vi "CRYPIC PreLoad.vi"(9 "sVIName":string) -> (1 "sVITitle_Out":string)   [LabVIEW 2013]
uses:
  DataView/VIEW/CRYView Global.vi
  CRYMain Sub Window Global.vi
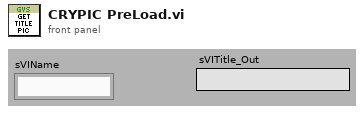
[diagram p1: front panel]
types:
  T1 = cluster{"sAction":string, "sType":string, "sQueueName":string, "sGraphName":string, "sData":string, "nData":i32, "pVIRef":refnum<vi>, "pSPRef":refnum<vi>}
  T2 = typedef "LVRectTypeDef.ctl" = cluster{"Left":i16, "Top":i16, "Right":i16, "Bottom":i16}
  T3 = cluster{"nType":i32, "nParent":i32, "pVIW":refnum<vi>, "pSPW":refnum<vi>, "nTypeF":i32, "pVIF":refnum<vi>, "pSPF":refnum<vi>, "nIDSpliter":i32, "nProperty":i32, "Bound":T2, "nID":i32, "nData":i32, "sData":string, "pWVI":refnum<vi>, "sTitle":string, "cPages":cluster{"nPage":i32, "sTitle":string, "sIcon":string, "pVI":refnum<vi>, "nID":i32}[], "pTab":refnum<vi>, "nIDPages":i32[], "pSPT":refnum<vi>, "sTemp":string, "nDockID":i32, "nDockLR":i32, "sIcon":string}
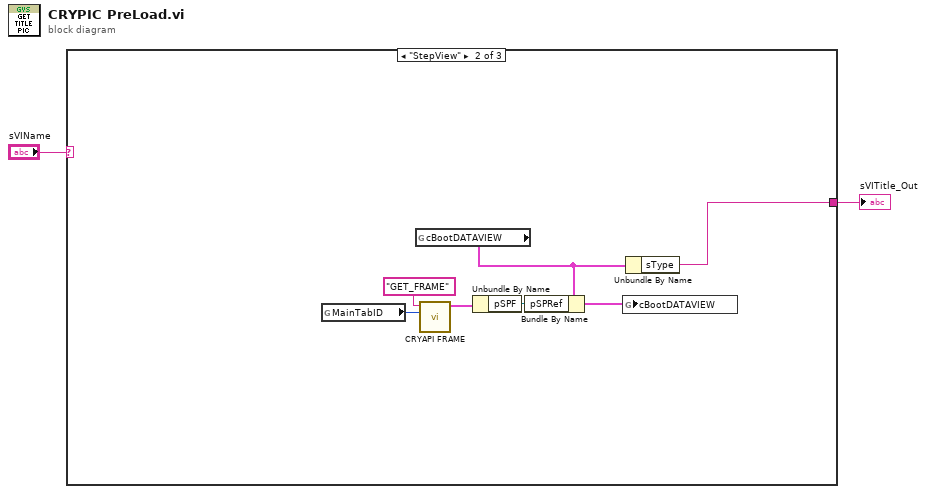
[diagram p0: block diagram]
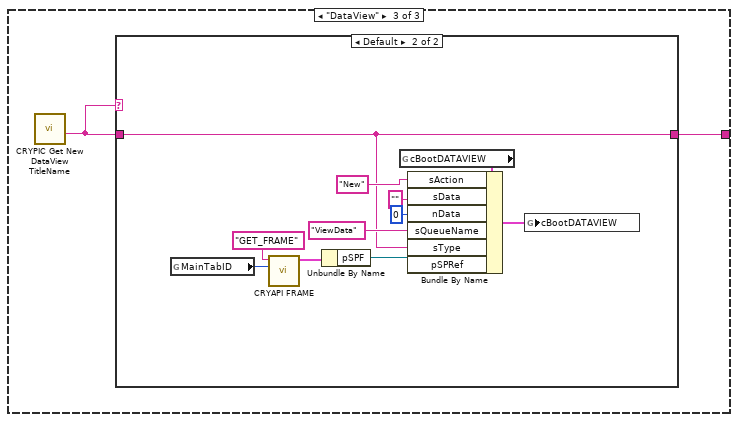
[diagram p3: hidden frame]
diagram:
  n1 = case shown="\"StepView\"" "sVIName" {
    selector: "sVIName" -> [w3 _ _]
    tunnel: [w3 w10 w12] -> w2
    frame Default {
    }
    frame "StepView" {
      n2 = global read "CRYMain Sub Window Global.vi" "MainTabID"() -> (w8:i32)
      n3 = global read "CRYView Global.vi" "cBootDATAVIEW"() -> (w7:T1)
      n4 = call "CRYAPI FRAME.vi"("nData"=w8, "sAction"="GET_FRAME") -> ("tFrame_Out"=w9:T3)  [unwired: 4 in, 5 out]
      n5 = Unbundle By Name(w9) -> ("pSPF"=w6:refnum<vi>)
      n6 = Bundle By Name(cluster=w7, "pSPRef"=w6) -> (w5:T1)
      n7 = global write "CRYView Global.vi" "cBootDATAVIEW"(w5) -> ()
      n8 = Unbundle By Name(w7) -> ("sType"=w10:string)
    }
    frame "DataView" {
      n9 = call "CRYPIC Get New DataView TitleName.vi"() -> ("sData_Out"=w11:string)  [unwired: 11 in]
      n10 = case shown="Default" w11 {
        tunnel: w11 -> [w13 w14]
        tunnel: [w13 w14] -> w12
        frame "" {
        }
        frame Default {
          n11 = global read "CRYMain Sub Window Global.vi" "MainTabID"() -> (w17:i32)
          n12 = call "CRYAPI FRAME.vi"("nData"=w17, "sAction"="GET_FRAME") -> ("tFrame_Out"=w16:T3)  [unwired: 4 in, 5 out]
          n13 = Unbundle By Name(w16) -> ("pSPF"=w15:refnum<vi>)
          n14 = global read "CRYView Global.vi" "cBootDATAVIEW"() -> (w20:T1)
          n15 = Bundle By Name(cluster=w20, "sAction"="New" ("sData"), "sData"="", "nData"=0, "sQueueName"="ViewData" ("sData"), "sType"=w14, "pSPRef"=w15) -> (w21:T1)
          n16 = global write "CRYView Global.vi" "cBootDATAVIEW"(w21) -> ()
        }
      }
    }
  }
  "sVITitle_Out" <- w2
